vi "LateUpdate.vi"(8 "error in (no error)":errorcluster, 11 "PongBall in":refnum<class "PongBall.lvclass">) -> (0 "error out":errorcluster, 3 "PongBall out":refnum<class "PongBall.lvclass">)   [LabVIEW 2019, in "RT_Game.lvlib" / "PongBall.lvclass"]
uses:
  PongBall.lvclass
  RT_Sprite/RT_Sprite.lvclass
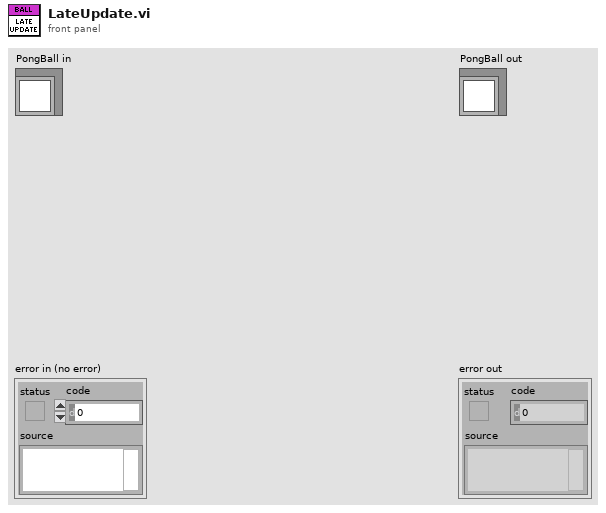
[diagram p1: front panel]
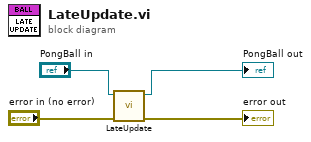
[diagram p0: block diagram]
diagram:
  n1 = call-parent "LateUpdate.vi"("error in (no error)"="error in (no error)", "GameObject in"="PongBall in") -> ("error out"=→"error out":errorcluster, "GameObject out"=→"PongBall out":refnum<class "PongBall.lvclass">)  [unwired: 8 in]
